vi "Get Style List.vi"(8 "error in (no error)":errorcluster, 11 "Document in":refnum<class "Document.lvclass">) -> (0 "error out":errorcluster, 2 "Style List":string[](array[string]), 3 "Document out":refnum<class "Document.lvclass">)   [LabVIEW 2017, in "LabVIEW NPOI.lvlib" / "Document.lvclass"]
uses:
  Document.lvclass
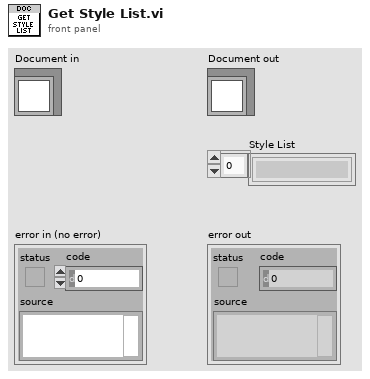
[diagram p1: front panel]
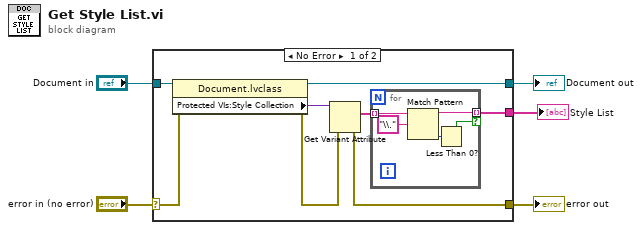
[diagram p0: block diagram]
diagram:
  n1 = case shown="No Error" "error in (no error)" {
    selector: "error in (no error)" -> [w11 w20]
    tunnel: [w8 w20] -> w4
    tunnel: [w12 w19] -> w2
    tunnel: "Document in" -> [w13 w19]
    tunnel: [w6 _] -> w1
    frame No Error {
      n2 = property class="Document.lvclass"(reference=w13, error in=w11) -> (reference out=w12:refnum<class "Document.lvclass">, error out=w9:errorcluster, "Protected VIs:Style Collection"=w10:variant)
      n3 = Get Variant Attribute(Variant=w10, error in=w9) -> (names=w7:string[], error out=w8:errorcluster)  [unwired: 2 in, 2 out]
      n4 = for {
        tunnel: w7 -> [w18] mode=indexing
        tunnel: [w16] -> w6 mode=indexing if=w15
        n5 = Match Pattern(string=w18, regular expression="\\.") -> (before substring=w16:string, offset past match=w14:i32)  [unwired: 1 in, 2 out]
        n6 = Less Than 0?(x=w14) -> (x < 0?=w15:bool)
      }
    }
    frame Error {
    }
  }
  "error out" <- w4
  "Document out" <- w2
  "Style List" <- w1
